vi "Write library name.vi"(8 "error in":errorcluster, 10 "library name":string, 11 "editorscriptingobject in":refnum<class "editorscriptingobjectadv.lvclass">) -> (0 "error out":errorcluster, 3 "editorscriptingobject out":refnum<class "editorscriptingobjectadv.lvclass">)   [LabVIEW 2015, in "editorscriptingobjectadv.lvclass"]
uses:
  editorscriptingobjectadv.lvclass
  editorscriptingobjectadv.lvclass/editorscriptingobjectadv.ctl
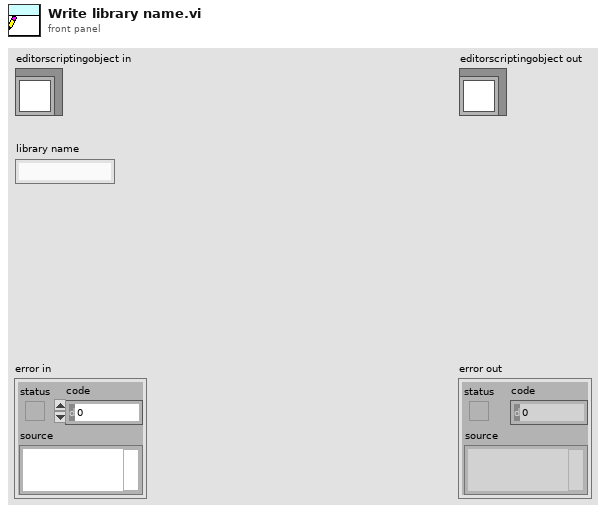
[diagram p1: front panel]
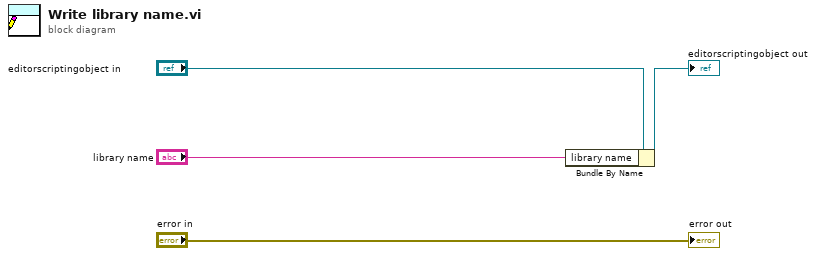
[diagram p0: block diagram]
diagram:
  n1 = Bundle By Name(cluster="editorscriptingobject in", "library name"="library name") -> (→"editorscriptingobject out":refnum<class "editorscriptingobjectadv.lvclass">)
  "error out" <- "error in"
